vi "Compile EPTx RevA Data.vi"(8 "error in (no error)":errorcluster, 10 "Compiled Data":T1 {"DI-B Injection"."Settings"."Pump Phase Array"."Profile" max=15; "DI-B Injection"."Settings"."Pump Phase Array"."Period [s]" min=0 max=0.000102 format="%#_3p"; "DI-B Injection"."Settings"."Pump Phase Array"."Pulse Width [s]" min=0 max=0.000102 format="%#_3p"; "DI-B Injection"."Settings"."Pump Phase Array"."Voltage Low [V]" min=-250 max=250 format="%#_3p"; "DI-B Injection"."Settings"."Pump Phase Array"."Voltage High [V]" min=-250 max=250 format="%#_3p"; "DI-B Injection"."Settings"."Pump Phase Array"."Current Low [A]" min=-40 max=40 format="%#_3p"; "DI-B Injection"."Settings"."Pump Phase Array"."Current High [A]" min=-40 max=40 format="%#_3p"; "DI-B Injection"."Settings"."Pump Phase Array"."Duration [s]" min=0 max=1.67772 format="%#_3p"; "DI-B Injection"."Settings"."Inj Phase Arrays"."Profile" max=15; "DI-B Injection"."Settings"."Inj Phase Arrays"."Period [s]" min=0 max=0.000102 format="%#_3p"; "DI-B Injection"."Settings"."Inj Phase Arrays"."Pulse Width [s]" min=0 max=0.000102 format="%#_3p"; "DI-B Injection"."Settings"."Inj Phase Arrays"."Voltage Low [V]" min=-250 max=250 format="%#_3p"; "DI-B Injection"."Settings"."Inj Phase Arrays"."Voltage High [V]" min=-250 max=250 format="%#_3p"; "DI-B Injection"."Settings"."Inj Phase Arrays"."Current Low [A]" min=-40 max=40 format="%#_3p"; "DI-B Injection"."Settings"."Inj Phase Arrays"."Current High [A]" min=-40 max=40 format="%#_3p"; "DI-B Injection"."Settings"."Inj Phase Arrays"."Duration [s]" min=0 max=1.67772 format="%#_3p"; "DI-A Injection"."Settings"."Pump Phase Array"."Profile" max=15; "DI-A Injection"."Settings"."Pump Phase Array"."Period [s]" min=0 max=0.000102 format="%#_3p"; "DI-A Injection"."Settings"."Pump Phase Array"."Pulse Width [s]" min=0 max=0.000102 format="%#_3p"; "DI-A Injection"."Settings"."Pump Phase Array"."Voltage Low [V]" min=-250 max=250 format="%#_3p"; "DI-A Injection"."Settings"."Pump Phase Array"."Voltage High [V]" min=-250 max=250 format="%#_3p"; "DI-A Injection"."Settings"."Pump Phase Array"."Current Low [A]" min=-40 max=40 format="%#_3p"; "DI-A Injection"."Settings"."Pump Phase Array"."Current High [A]" min=-40 max=40 format="%#_3p"; "DI-A Injection"."Settings"."Pump Phase Array"."Duration [s]" min=0 max=1.67772 format="%#_3p"; "DI-A Injection"."Settings"."Inj Phase Arrays"."Profile" max=15; "DI-A Injection"."Settings"."Inj Phase Arrays"."Period [s]" min=0 max=0.000102 format="%#_3p"; "DI-A Injection"."Settings"."Inj Phase Arrays"."Pulse Width [s]" min=0 max=0.000102 format="%#_3p"; "DI-A Injection"."Settings"."Inj Phase Arrays"."Voltage Low [V]" min=-250 max=250 format="%#_3p"; "DI-A Injection"."Settings"."Inj Phase Arrays"."Voltage High [V]" min=-250 max=250 format="%#_3p"; "DI-A Injection"."Settings"."Inj Phase Arrays"."Current Low [A]" min=-40 max=40 format="%#_3p"; "DI-A Injection"."Settings"."Inj Phase Arrays"."Current High [A]" min=-40 max=40 format="%#_3p"; "DI-A Injection"."Settings"."Inj Phase Arrays"."Duration [s]" min=0 max=1.67772 format="%#_3p"; "Knock"."Settings"."Sensor Select" items=["Sensor 1", "Sensor 2", "Sensor 3", "Sensor 4", "Sensor 5", "Sensor 6", "Sensor 7", "Sensor 8", "Sensor 9", "Sensor 10", "Sensor 11", "Sensor 12"]; "PBx"."PB-01"."FIFO Indexes"."Read"."UEGO Diagnostics"."LSUType" format="%02.0f"; "PBx"."PB-01"."FIFO Indexes"."Read"."UEGO Diagnostics"."UEGOFuseStatus" format="%02.0f"; "DCM Core"."Settings"."System Settings"."HH Open Threshold [A]" min=0 max=8 format="%#_3p"; "DCM Core"."Settings"."System Settings"."HH ISeq Dur PS" items=["3.3ms @ 20MHz"=0, "6.5ms @ 10MHz"=4, "13ms @ 5MHz"=6, "26ms @ 2.5MHz"=7]; "DCM Core"."Settings"."System Settings"."HH Shoot Through Time [s]" min=0 max=0.003277 format="%#_3p"; "DCM Core"."Settings"."System Settings"."Clamp Fault Filter Time [s]" min=0 max=0.003277 format="%#_3p"; "DCM Core"."Settings"."System Settings"."DI HS Fault Filter Time [s]" min=0 max=0.003277 format="%#_3p"; "DCM Core"."Settings"."B Configuration"."Pump Zener Voltage [V]" min=0 max=240 format="%#_13g"; "DCM Core"."Settings"."B Configuration"."DI Zener Voltage [V]" min=0 max=100 format="%#_13g"; "DCM Core"."Settings"."B Configuration"."Boost Clamp [V]" min=0 max=220 format="%#_13g"; "DCM Core"."Settings"."B Configuration"."Boost Voltage [V]" min=0 max=220 format="%#_13g"; "DCM Core"."Settings"."A Configuration"."Pump Zener Voltage [V]" min=0 max=240 format="%#_13g"; "DCM Core"."Settings"."A Configuration"."DI Zener Voltage [V]" min=0 max=100 format="%#_13g"; "DCM Core"."Settings"."A Configuration"."Boost Clamp [V]" min=0 max=220 format="%#_13g"; "DCM Core"."Settings"."A Configuration"."Boost Voltage [V]" min=0 max=220 format="%#_13g"; "DCM Core"."FIFO Indexes"."Write"."HH Config"."ISeq"."Duration [s]" min=0 max=26; "DCM Core"."FIFO Indexes"."Write"."HH Config"."ISeq"."Lower [A]" min=0 max=8; "DCM Core"."FIFO Indexes"."Write"."HH Config"."ISeq"."Upper [A]" min=0 max=8; "Digital Signals"."Settings"."Aux In Filters [s]" min=0; "Digital Signals"."Settings"."Diff IO Filters [s]" min=0; "EPTx RevA"."Settings"."EPTxFilters"."Aux 4 [s]" format="%#_6p"; "EPTx RevA"."Settings"."EPTxFilters"."Aux 3 [s]" format="%#_6p"; "EPTx RevA"."Settings"."EPTxFilters"."Aux 2 [s]" format="%#_6p"; "EPTx RevA"."Settings"."EPTxFilters"."Aux 1 [s]" format="%#_6p"; "EPTx RevA"."Settings"."EPTxFilters"."Primary [s]" format="%#_6p"}, 11 "Device Item Ref in":T40 format="%.0x") -> (0 "error out":errorcluster, 2 "Compiled Data":T1 {"DI-B Injection"."Settings"."Pump Phase Array"."Profile" max=15; "DI-B Injection"."Settings"."Pump Phase Array"."Period [s]" min=0 max=0.000102 format="%#_3p"; "DI-B Injection"."Settings"."Pump Phase Array"."Pulse Width [s]" min=0 max=0.000102 format="%#_3p"; "DI-B Injection"."Settings"."Pump Phase Array"."Voltage Low [V]" min=-250 max=250 format="%#_3p"; "DI-B Injection"."Settings"."Pump Phase Array"."Voltage High [V]" min=-250 max=250 format="%#_3p"; "DI-B Injection"."Settings"."Pump Phase Array"."Current Low [A]" min=-40 max=40 format="%#_3p"; "DI-B Injection"."Settings"."Pump Phase Array"."Current High [A]" min=-40 max=40 format="%#_3p"; "DI-B Injection"."Settings"."Pump Phase Array"."Duration [s]" min=0 max=1.67772 format="%#_3p"; "DI-B Injection"."Settings"."Inj Phase Arrays"."Profile" max=15; "DI-B Injection"."Settings"."Inj Phase Arrays"."Period [s]" min=0 max=0.000102 format="%#_3p"; "DI-B Injection"."Settings"."Inj Phase Arrays"."Pulse Width [s]" min=0 max=0.000102 format="%#_3p"; "DI-B Injection"."Settings"."Inj Phase Arrays"."Voltage Low [V]" min=-250 max=250 format="%#_3p"; "DI-B Injection"."Settings"."Inj Phase Arrays"."Voltage High [V]" min=-250 max=250 format="%#_3p"; "DI-B Injection"."Settings"."Inj Phase Arrays"."Current Low [A]" min=-40 max=40 format="%#_3p"; "DI-B Injection"."Settings"."Inj Phase Arrays"."Current High [A]" min=-40 max=40 format="%#_3p"; "DI-B Injection"."Settings"."Inj Phase Arrays"."Duration [s]" min=0 max=1.67772 format="%#_3p"; "DI-A Injection"."Settings"."Pump Phase Array"."Profile" max=15; "DI-A Injection"."Settings"."Pump Phase Array"."Period [s]" min=0 max=0.000102 format="%#_3p"; "DI-A Injection"."Settings"."Pump Phase Array"."Pulse Width [s]" min=0 max=0.000102 format="%#_3p"; "DI-A Injection"."Settings"."Pump Phase Array"."Voltage Low [V]" min=-250 max=250 format="%#_3p"; "DI-A Injection"."Settings"."Pump Phase Array"."Voltage High [V]" min=-250 max=250 format="%#_3p"; "DI-A Injection"."Settings"."Pump Phase Array"."Current Low [A]" min=-40 max=40 format="%#_3p"; "DI-A Injection"."Settings"."Pump Phase Array"."Current High [A]" min=-40 max=40 format="%#_3p"; "DI-A Injection"."Settings"."Pump Phase Array"."Duration [s]" min=0 max=1.67772 format="%#_3p"; "DI-A Injection"."Settings"."Inj Phase Arrays"."Profile" max=15; "DI-A Injection"."Settings"."Inj Phase Arrays"."Period [s]" min=0 max=0.000102 format="%#_3p"; "DI-A Injection"."Settings"."Inj Phase Arrays"."Pulse Width [s]" min=0 max=0.000102 format="%#_3p"; "DI-A Injection"."Settings"."Inj Phase Arrays"."Voltage Low [V]" min=-250 max=250 format="%#_3p"; "DI-A Injection"."Settings"."Inj Phase Arrays"."Voltage High [V]" min=-250 max=250 format="%#_3p"; "DI-A Injection"."Settings"."Inj Phase Arrays"."Current Low [A]" min=-40 max=40 format="%#_3p"; "DI-A Injection"."Settings"."Inj Phase Arrays"."Current High [A]" min=-40 max=40 format="%#_3p"; "DI-A Injection"."Settings"."Inj Phase Arrays"."Duration [s]" min=0 max=1.67772 format="%#_3p"; "Knock"."Settings"."Sensor Select" items=["Sensor 1", "Sensor 2", "Sensor 3", "Sensor 4", "Sensor 5", "Sensor 6", "Sensor 7", "Sensor 8", "Sensor 9", "Sensor 10", "Sensor 11", "Sensor 12"]; "PBx"."PB-01"."FIFO Indexes"."Read"."UEGO Diagnostics"."LSUType" format="%02.0f"; "PBx"."PB-01"."FIFO Indexes"."Read"."UEGO Diagnostics"."UEGOFuseStatus" format="%02.0f"; "DCM Core"."Settings"."System Settings"."HH Open Threshold [A]" min=0 max=8 format="%#_3p"; "DCM Core"."Settings"."System Settings"."HH ISeq Dur PS" items=["3.3ms @ 20MHz"=0, "6.5ms @ 10MHz"=4, "13ms @ 5MHz"=6, "26ms @ 2.5MHz"=7]; "DCM Core"."Settings"."System Settings"."HH Shoot Through Time [s]" min=0 max=0.003277 format="%#_3p"; "DCM Core"."Settings"."System Settings"."Clamp Fault Filter Time [s]" min=0 max=0.003277 format="%#_3p"; "DCM Core"."Settings"."System Settings"."DI HS Fault Filter Time [s]" min=0 max=0.003277 format="%#_3p"; "DCM Core"."Settings"."B Configuration"."Pump Zener Voltage [V]" min=0 max=240 format="%#_13g"; "DCM Core"."Settings"."B Configuration"."DI Zener Voltage [V]" min=0 max=100 format="%#_13g"; "DCM Core"."Settings"."B Configuration"."Boost Clamp [V]" min=0 max=220 format="%#_13g"; "DCM Core"."Settings"."B Configuration"."Boost Voltage [V]" min=0 max=220 format="%#_13g"; "DCM Core"."Settings"."A Configuration"."Pump Zener Voltage [V]" min=0 max=240 format="%#_13g"; "DCM Core"."Settings"."A Configuration"."DI Zener Voltage [V]" min=0 max=100 format="%#_13g"; "DCM Core"."Settings"."A Configuration"."Boost Clamp [V]" min=0 max=220 format="%#_13g"; "DCM Core"."Settings"."A Configuration"."Boost Voltage [V]" min=0 max=220 format="%#_13g"; "DCM Core"."FIFO Indexes"."Write"."HH Config"."ISeq"."Duration [s]" min=0 max=26; "DCM Core"."FIFO Indexes"."Write"."HH Config"."ISeq"."Lower [A]" min=0 max=8; "DCM Core"."FIFO Indexes"."Write"."HH Config"."ISeq"."Upper [A]" min=0 max=8; "Digital Signals"."Settings"."Aux In Filters [s]" min=0; "Digital Signals"."Settings"."Diff IO Filters [s]" min=0; "EPTx RevA"."Settings"."EPTxFilters"."Aux 4 [s]" format="%#_6p"; "EPTx RevA"."Settings"."EPTxFilters"."Aux 3 [s]" format="%#_6p"; "EPTx RevA"."Settings"."EPTxFilters"."Aux 2 [s]" format="%#_6p"; "EPTx RevA"."Settings"."EPTxFilters"."Aux 1 [s]" format="%#_6p"; "EPTx RevA"."Settings"."EPTxFilters"."Primary [s]" format="%#_6p"}, 3 "Device Item Ref out":T40 format="%.0x")   [LabVIEW 2016, in "DCM System Explorer.lvlib"]
uses:
  DCM System Explorer.lvlib
  <vilib>/NI Veristand/Custom Device API/Custom Device Item Ref.ctl
  Shared/Types/Compiled Data.ctl
  <vilib>/NI Veristand/Custom Device Waveform API/Multiple Waveforms Write (DBL)/Multiple Waveforms Write (DBL).lvclass
  Shared/Types/Engine Init Data.ctl
  Shared/Types/Engine Status.ctl
  Shared/Types/EPTx RevA RT Data.ctl
  Built/DCM Classes Packed/Pharlap/C/DCM-Classes.lvlibp/1abvi3w/vi.lib/Powertrain Controls/Device Drivers/DCM/Rev0/FPGA/Digital Channel.ctl
  Built/DCM Classes Packed/Pharlap/C/DCM-Classes.lvlibp/Engine Position Tracking/EPTx/RevA/RT/Controls/EPTxFilters.ctl
  Shared/Types/DCM Core.ctl
  Shared/Types/System State Indexes.ctl
  Shared/Types/DI Faults Indexes.ctl
  Shared/Types/HH Status Indexes.ctl
  Shared/Types/HH Config Indexes.ctl
  <vilib>/Powertrain Controls/Device Drivers/DCM/Rev0/RT/Configuration.ctl
  <vilib>/Powertrain Controls/Device Drivers/DCM/Rev0/FPGA/DI - Bank Configuration.ctl
  <vilib>/Powertrain Controls/Device Drivers/DCM/Rev0/RT/System Settings.ctl
  <vilib>/Powertrain Controls/Device Drivers/DCM/Rev0/RT/User LED.ctl
  <vilib>/Powertrain Controls/Device Drivers/DCM/HH/RT/Duration Pre Scale.ctl
  Shared/Types/DI.ctl
  Shared/Types/DI Command Indexes.ctl
  Shared/Types/DI Phase Outputs.ctl
  <vilib>/Powertrain Controls/Device Drivers/DCM/DI/RT/Phase.ctl
  <vilib>/Powertrain Controls/Device Drivers/DCM/Rev0/FPGA/DI - Drive State.ctl
  <vilib>/Powertrain Controls/Device Drivers/DCM/DI/FPGA/Phase Step.ctl
  <vilib>/Powertrain Controls/Device Drivers/DCM/DI/FPGA/Control.ctl
  Shared/Types/DiffIO.ctl
  Shared/Types/DiffIO Results Indexes.ctl
  Shared/Types/DiffIO Setup Indexes.ctl
  Shared/Types/HH.ctl
  Shared/Types/HH Command Indexes.ctl
  Shared/Types/DI Scope.ctl
  <vilib>/NI Veristand/Custom Device API/Waveform Data Reference.ctl
  Shared/Types/HH Scope.ctl
  Shared/Types/Digital Signals.ctl
  Shared/Types/Skip Fire.ctl
  Shared/Types/Skip Fire Setup Indexes.ctl
  Shared/Types/Knock.ctl
  Shared/Types/PBx.ctl
  Shared/Types/PB-01.ctl
  Shared/Types/ESTTL Setup Indexes.ctl
  <vilib>/Powertrain Controls/Device Drivers/VR-Hall/RevC/Real-Time/Support/Vr_Hall_mode_control_revc.ctl
  Shared/Types/EPTx Signal Select.ctl
  <vilib>/Powertrain Controls/Device Drivers/DCM/Rev0/FPGA/Digital Channel.ctl
  Shared/Types/EPTx RevA RT Configuration.ctl
  <vilib>/Powertrain Controls/Device Drivers/Engine Position Tracking/EPTx/RevA/RT/Controls/EPTxFilters.ctl
  Shared/DCM Properties.vi
  Shared/DCM Constants and GUIDs.vi
  <vilib>/NI Veristand/Custom Device Tools/Custom Device Utility Library/NI VeriStand - Search for Item by GUID.vi
  <vilib>/NI Veristand/Custom Device Tools/Custom Device Utility Library/Custom Device Utility Library.lvlib
  DCM Shared.lvlib
  <vilib>/Powertrain Controls/Device Drivers/DCM/Rev0/FPGA/DCM - FPGA.lvlib
  <vilib>/Powertrain Controls/Device Drivers/Engine Position Tracking/EPTx/RevA/RT/EPTx - RevA - RT.lvlib
  <vilib>/NI VeriStand/Custom Device API/Custom Device API.lvlib
  <vilib>/Powertrain Controls/Device Drivers/DCM/Rev0/RT/DCM - RT.lvclass
  <vilib>/Powertrain Controls/Device Drivers/DCM/HH/RT/DCM - RT - HH.lvlib
  <vilib>/Powertrain Controls/Device Drivers/DCM/DI/FPGA/DCM - FPGA - DI.lvlib
  <vilib>/Powertrain Controls/Device Drivers/DCM/DI/RT/DCM - RT - DI.lvlib
  Built/DCM Classes Packed/Pharlap/C/DCM-Classes.lvlibp/Engine Position Tracking/EPTx/RevA/RT/EPTx - RevA - RT.lvlib
  Built/DCM Classes Packed/Pharlap/C/DCM-Classes.lvlibp/1abvi3w/vi.lib/Powertrain Controls/Device Drivers/DCM/Rev0/FPGA/DCM - FPGA.lvlib
panel:
  # "Voltage [DV]"
  # "Voltage [V]"
  # "Voltage [DV]"
  # "Voltage [V]"
  # "Voltage [DV]"
  # "Voltage [V]"
  # "Voltage [DV]"
  # "Voltage [V]"
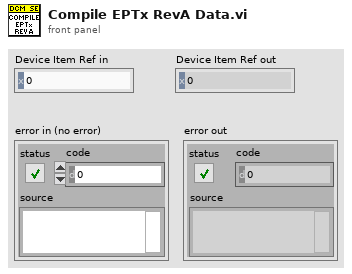
[diagram p1: front panel]
types:
  T1 = typedef "DCM Shared.lvlib/Compiled Data.ctl" = cluster{"Init":T2, "Cmd Status":T3, "Sys Status":T3, "EPTx RevA":T4, "DCM Core":T7, "DI-A Injection":T17, "DI-B Injection":T17, "DiffIO":T24, "HH Cmd":T27, "DI ADC":T29, "HH ADC":T31, "Digital Signals":T32, "Skip Fire":T33, "Knock":T35, "PBx":T36}
  T2 = typedef "DCM Shared.lvlib/Engine Init Data.ctl" = cluster{"Name":string, "RIO Address":string, "Bitfile Path RT":path, "Username":string, "Password":string, "Cmd CPU":i32, "Cmd Decimation":i32, "Cmd Priority":i32, "Sys CPU":i32, "Sys Decimation":i32, "Sys Priority":i32, "Input FIFO Size":i32, "Output FIFO Size":i32, "Compile Time":dbl}
  T3 = typedef "DCM Shared.lvlib/Engine Status.ctl" = cluster{"FIFO indexes":cluster{"code":i32, "loop duration":i32, "late count":i32}}
  T4 = typedef "DCM Shared.lvlib/EPTx RevA RT Data.ctl" = cluster{"FIFO Indexes":cluster{"Read":cluster{"Sync":i32, "CurrentCAD":i32, "Speed":i32, "Config":i32, "Rcvg Primary":i32, "Stall":i32, "Overflow Error":i32, "Ratio Error":i32, "Pattern Error":i32, "Aux Warning":i32, "Watchdog Error":i32, "Loading":i32}, "Write":cluster{"Reload EPTx":i32, "Sync Enable":i32, "Clear Errors":i32, "Sim Enable":i32, "Sim Speed":i32}}, "Settings":cluster{"EPTxConfigFilename":string, "EPTx Signal Select":cluster{"Primary":T5, "Aux 1":T5, "Aux 2":T5, "Aux 3":T5, "Aux 4":T5}, "FPGAFrequency":sgl, "StallSpeed":sgl, "EPTxFilters":T6, "History":u8}}
  T5 = typedef "DCM-Classes.lvlibp/DCM - FPGA.lvlib/Digital Channel.ctl" = enum8{"Unused", "User OS", "Diff IO 1", "Diff IO 2", "Diff IO 3", "Diff IO 4", "Diff IO 5", "Diff IO 6", "Diff IO 7", "Diff IO 8", "Aux 1", "Aux 2", "Aux 3", "Aux 4", "Aux 5", "Aux 6", "Aux 7", "Aux 8", "Aux 9", "Aux 10", "Aux 11", "Aux 12", "Aux 13", "Aux 14", "Aux 15", "Aux 16"}
  T6 = typedef "DCM-Classes.lvlibp/EPTx - RevA - RT.lvlib/EPTxFilters.ctl" = cluster{"Primary [s]":sgl, "Aux 1 [s]":sgl, "Aux 2 [s]":sgl, "Aux 3 [s]":sgl, "Aux 4 [s]":sgl}
  T7 = typedef "DCM Shared.lvlib/DCM Core.ctl" = cluster{"FIFO Indexes":cluster{"A Run State":i32, "B Run State":i32, "Read":cluster{"Status":T8, "A DI Faults":T9[], "B DI Faults":T9[], "HH Status":T10[]}, "Write":cluster{"A Config":cluster{"PowerSupplyEnable":i32, "InjectEnable":i32, "BoostVoltage":i32}, "B Config":cluster{"PowerSupplyEnable":i32, "InjectEnable":i32, "BoostVoltage":i32}, "HH Config":T11[], "System Settings":cluster{"MPRD":i32, "UserLED1":i32, "UserLED2":i32}, "A Fault Clear":cluster{"1":i32, "2":i32, "3":i32, "4":i32, "5":i32, "6":i32, "7":i32, "8":i32}, "B Fault Clear":cluster{"1":i32, "2":i32, "3":i32, "4":i32, "5":i32, "6":i32, "7":i32, "8":i32}}}, "Settings":cluster{"A Configuration":T12, "B Configuration":T12, "System Settings":T14}}
  T8 = typedef "DCM Shared.lvlib/System State Indexes.ctl" = cluster{"System ADC":cluster{"AI 1 [V]":i32, "AI 2 [V]":i32, "AI 3 [V]":i32, "AI 4 [V]":i32, "AI 5 [V]":i32, "AI 6 [V]":i32, "AI 7 [V]":i32, "AI 8 [V]":i32, "AI 9 [V]":i32, "AI 10 [V]":i32, "AI 11 [V]":i32, "AI 12 [V]":i32, "Temp HH 1-6 [C]":i32, "Temp HH 7-12 [C]":i32, "Temp DI A [C]":i32, "Temp DI Zener A [C]":i32, "Temp DI B [C]":i32, "Temp DI Zener B [C]":i32, "Temp CPU [C]":i32, "Temp Fan Intake [C]":i32, "Temp Secondary A [C]":i32, "Temp Primary A [C]":i32, "Temp Boost B [C]":i32, "Primary Range [V]":i32, "Primary A1A2 [V]":i32, "Primary A3A4 [V]":i32, "Primary B3B4 [V]":i32, "Primary B1B2 [V]":i32, "Secondary A1A2 [V]":i32, "Secondary A3A4 [V]":i32, "Secondary B3B4 [V]":i32, "Secondary B1B2 [V]":i32, "Ext HV A [V]":i32, "Ext HV B [V]":i32, "FET Driver [V]":i32, "Fan [V]":i32, "Battery [V]":i32, "DRVP [V]":i32, "Key [V]":i32, "DI Zener A [V]":i32, "DI Zener B [V]":i32, "Pump Zener A [V]":i32, "Pump Zener B [V]":i32, "MPRD [V]":i32}, "IO Lock":i32, "HH Mode Config Error":i32, "Fan Speed 1 [RPM]":i32, "Fan Speed 2 [RPM]":i32, "Firmware Major Rev":i32, "Firmware Minor Rev":i32, "Internal Fault":i32, "Fault Value":i32}
  T9 = typedef "DCM Shared.lvlib/DI Faults Indexes.ctl" = cluster{"HV Fault":i32, "LV Fault":i32, "LS Fault":i32, "MUX Fault":i32, "Open Warning":i32}
  T10 = typedef "DCM Shared.lvlib/HH Status Indexes.ctl" = cluster{"Current [A]":i32, "Config Error":i32, "Short Fault":i32, "Open Fault":i32, "Period Min [A]":i32, "Period Max [A]":i32, "Period Avg [A]":i32, "On Avg [A]":i32}
  T11 = typedef "DCM Shared.lvlib/HH Config Indexes.ctl" = cluster{"Mode":i32, "IO Lock State":i32, "Phase 1 FP":i32, "Fault Clear":i32, "ISeq":cluster{"Upper [A]":i32, "Lower [A]":i32, "Duration [s]":i32}[]}
  T12 = typedef "DCM - RT.lvclass/Configuration.ctl" = cluster{"Configuration":T13, "Power Supply Enable":bool, "Boost Voltage [V]":sgl, "Inject Enable":bool, "DI Zener Enable":bool, "DI Zener Voltage [V]":sgl, "Pump Zener Enable":bool, "Pump Zener Voltage [V]":sgl, "Boost Clamp [V]":sgl}
  T13 = typedef "DCM - FPGA.lvlib/DI - Bank Configuration.ctl" = enum8{"Solenoid Unipolar 4", "Solenoid Unipolar 7 (Muxed)", "Solenoid Unipolar 8 (Muxed)", "Solenoid Bipolar 2", "Solenoid Bipolar 3 (Muxed)", "Piezo Unipolar 2", "Piezo Unipolar 3 (Muxed)", "Piezo Unipolar 4 (Muxed)", "Piezo Bipolar 2", "Piezo Bipolar 3 (Muxed)"}
  T14 = typedef "DCM - RT.lvclass/System Settings.ctl" = cluster{"MPRD":bool, "IO Lock MPRD Disable":bool, "User LED 1":T15, "User LED 2":T15, "DI HS Fault Filter Time [s]":sgl, "Clamp Fault Filter Time [s]":sgl, "HH Shoot Through Time [s]":sgl, "HH ISeq Dur PS":T16, "HH Open Threshold [A]":sgl}
  T15 = typedef "DCM - RT.lvclass/User LED.ctl" = enum16{"Off", "Yellow", "Green"}
  T16 = typedef "DCM - RT - HH.lvlib/Duration Pre Scale.ctl" = u8
  T17 = typedef "DCM Shared.lvlib/DI.ctl" = cluster{"DI Command Enabled":bool, "Sync Pump Enabled":bool, "FIFO Indexes":cluster{"Write":cluster{"DI Command":T18[], "Pump Command":T18}}, "Settings":T19}
  T18 = typedef "DCM Shared.lvlib/DI Command Indexes.ctl" = cluster{"Mode":i32, "Digital Input":i32, "Default Profile Index":i32, "Cal Freq [Hz]":i32, "Cal Duration [s]":i32, "Cal Increment [s]":i32, "Cal Pulses":i32, "TMP Command Sequence":cluster{"Duration [s]":i32, "Level":i32, "Run/Stop":i32, "Profile Index":i32}[], "EPT TDC Offset [CAD]":i32, "EPT Window Start [DBTDC]":i32, "EPT Window End [DBTDC]":i32, "EPT Angles":cluster{"Enable":i32, "Timing [DBTDC]":i32, "Duration [s]":i32, "Profile Index":i32}[], "EPT Skip Fire":i32, "EPT Skip Index":i32, "EPT Precharge Duration [s]":i32, "EPT Precharge Profile Index":i32}
  T19 = typedef "DCM Shared.lvlib/DI Phase Outputs.ctl" = cluster{"Inj Phase Arrays":T20[][], "Pump Phase Array":T20[], "Pulsewidths [s]":sgl[][]}
  T20 = typedef "DCM - RT - DI.lvlib/Phase.ctl" = cluster{"Drive":T21, "Direction":bool, "Phase Step":T22, "Duration [s]":sgl, "Current High [A]":sgl, "Current Low [A]":sgl, "Voltage High [V]":sgl, "Voltage Low [V]":sgl, "Change":bool, "Current Control":T23, "Period [s]":sgl, "Pulse Width [s]":sgl, "Profile":u8, "Voltage Control":bool}
  T21 = typedef "DCM - FPGA.lvlib/DI - Drive State.ctl" = enum8{"Idle", "HV Current Control", "LV Current Control", "Back Boost", "Piezo Charge", "Piezo Discharge"}
  T22 = typedef "DCM - FPGA - DI.lvlib/Phase Step.ctl" = enum8{"Duration", "First Peak", "End of Cmd", "Branch", "2-Phase Duration"}
  T23 = typedef "DCM - FPGA - DI.lvlib/Control.ctl" = enum8{"Closed Loop", "Fixed Period", "Fixed On Pulse", "Fixed Off Pulse", "Open Loop", "Profile"}
  T24 = typedef "DCM Shared.lvlib/DiffIO.ctl" = cluster{"DiffIO Command Enabled":bool, "FIFO Indexes":cluster{"Read":cluster{"Diff IO Results":T25[], "DiffIOIn":cluster{"1":i32, "2":i32, "3":i32, "4":i32, "5":i32, "6":i32, "7":i32, "8":i32}}, "Write":cluster{"Diff I/O Setup":T26[]}}}
  T25 = typedef "DCM Shared.lvlib/DiffIO Results Indexes.ctl" = cluster{"Capture [DBTDC]":i32, "Capture Error":i32, "Frequency [Hz]":i32, "Duty Cycle [%]":i32, "PWM Stopped":i32}
  T26 = typedef "DCM Shared.lvlib/DiffIO Setup Indexes.ctl" = cluster{"Mode":i32, "Capture Start [DBTDC]":i32, "Capture End [DBTDC]":i32, "Polarity":i32, "Frequency [Hz]":i32, "Duty Cycle [%]":i32, "TDC Offset [CAD]":i32, "Window Start [DBTDC]":i32, "Window End [DBTDC]":i32, "Angles":cluster{"Enable":i32, "Location [DBTDC]":i32, "Duration [s]":i32}[], "Skip Fire":i32, "Skip Fire Index":i32}
  T27 = typedef "DCM Shared.lvlib/HH.ctl" = cluster{"HH Command Enabled":bool, "FIFO Indexes":cluster{"Write":T28[]}}
  T28 = typedef "DCM Shared.lvlib/HH Command Indexes.ctl" = cluster{"Mode":i32, "Digital Input":i32, "Polarity":i32, "Frequency [Hz]":i32, "Duty Cycle [%]":i32, "TDC Offset [CAD]":i32, "Window Start [DBTDC]":i32, "Window End [DBTDC]":i32, "Angles":cluster{"Enable":i32, "Location [DBTDC]":i32, "Duration [s]":i32}[], "Skip Fire":i32, "Skip Fire Index":i32}
  T29 = typedef "DCM Shared.lvlib/DI Scope.ctl" = cluster{"FIFO Indexes":cluster{"Write":cluster{"Capture Enable":i32, "Capture Event":i32, "Capture Length":i32, "DI ADC 1 Select":i32, "DI ADC 2 Select":i32, "DI ADC 3 Select":i32, "DI ADC 4 Select":i32}, "Read":cluster{"Capture dt [s]":i32}}, "DI ADC Data":cluster{"Output Array":sgl[][], "New Data":bool}, "Waveform Data":T30[], "Waveform Session":refnum<class "Multiple Waveforms Write (DBL).lvclass">}
  T30 = typedef "Custom Device API.lvlib/Waveform Data Reference.ctl" = i32
  T31 = typedef "DCM Shared.lvlib/HH Scope.ctl" = cluster{"FIFO Indexes":cluster{"Write":cluster{"Capture Enable":i32, "Capture Event":i32, "Capture Length":i32}, "Read":cluster{"Capture dt [s]":i32}}, "HH ADC Data":cluster{"Output Array":sgl[][], "New Data":bool}, "Waveform Data":T30[], "Waveform Session":refnum<class "Multiple Waveforms Write (DBL).lvclass">}
  T32 = typedef "DCM Shared.lvlib/Digital Signals.ctl" = cluster{"FIFO Indexes":cluster{"Write":cluster{"User OS":i32, "User OS Time [s]":i32}}, "Settings":cluster{"Diff IO Filters [s]":sgl[], "Aux In Filters [s]":sgl[]}}
  T33 = typedef "DCM Shared.lvlib/Skip Fire.ctl" = cluster{"Skip Fire Enabled":bool, "FIFO Indexes":cluster{"Write":cluster{"Setup":T34[]}}}
  T34 = typedef "DCM Shared.lvlib/Skip Fire Setup Indexes.ctl" = cluster{"Enable":i32, "Total Cycles":i32, "On Cycles":i32, "TDC Offset [CAD]":i32}
  T35 = typedef "DCM Shared.lvlib/Knock.ctl" = cluster{"FIFO Indexes":cluster{"Read":cluster{"Knock":i32[], "Knock Intensity":i32[]}, "Write":cluster{"Low Cutoff [Hz]":i32, "High Cutoff [Hz]":i32, "Threshold":i32, "Knock Start [CAD]":i32, "Knock End [CAD]":i32, "Reference Start [CAD]":i32, "Reference End [CAD]":i32}}, "Settings":cluster{"Sensor Select":i32[], "Cylinder Offset [CAD]":sgl[]}}
  T36 = typedef "DCM Shared.lvlib/PBx.ctl" = cluster{"PB Version":u8, "PB-01":T37}
  T37 = typedef "DCM Shared.lvlib/PB-01.ctl" = cluster{"FIFO Indexes":cluster{"Write":cluster{"Clear Faults":i32, "ESTTL Setup":T38[], "UEGO Control":cluster{"UEGO1Enable":i32, "UEGO2Enable":i32, "UEGO1Range":i32, "UEGO2Range":i32, "FilterCutoff (Hz)":i32}}, "Read":cluster{"UEGO Sensor Results":cluster{"UEGO1Lambda":i32, "UEGO1Phi":i32, "UEGO1AFRatio":i32, "UEGO1Ip (mA)":i32, "UEGO2Lambda":i32, "UEGO2Phi":i32, "UEGO2AFRatio":i32, "UEGO2Ip (mA)":i32}, "UEGO Temperature (C)":cluster{"UEGO1Temp (C)":i32, "UEGO2Temp (C)":i32, "UEGO1Hot":i32, "UEGO2Hot":i32}, "UEGO Diagnostics":cluster{"UEGO1SensorFault":i32, "UEGO2SensorFault":i32, "UEGO1HeaterFault":i32, "UEGO2HeaterFault":i32, "UEGOFuseStatus":i32, "Battery (V)":i32, "LSUType":i32}}}, "Settings":cluster{"VR-Hall Mode Select":T39[], "VR-Hall Arming Threshold [V]":dbl[], "ESTTL Command Enabled":bool}}
  T38 = typedef "DCM Shared.lvlib/ESTTL Setup Indexes.ctl" = cluster{"Mode":i32, "Polarity":i32, "Frequency [Hz]":i32, "Duty Cycle [%]":i32, "TDC Offset [CAD]":i32, "Window Start [DBTDC]":i32, "Window End [DBTDC]":i32, "Angles":cluster{"Enable":i32, "Location [DBTDC]":i32, "Duration [s]":i32}[], "Skip Fire":i32, "Skip Fire Index":i32}
  T39 = typedef "Vr_Hall_mode_control_revc.ctl" = enum32{"VR Adaptive Arm", "VR Manual Arm", "Hall", "Hall w/ Pull-up"}
  T40 = typedef "Custom Device API.lvlib/Custom Device Item Ref.ctl" = u64
  T41 = typedef "DCM Shared.lvlib/EPTx RevA RT Configuration.ctl" = cluster{"EPTx Configuration Filename":string, "StallSpeed":dbl, "HistoryCAD":u8, "EPTxFilters":T42}
  T42 = typedef "EPTx - RevA - RT.lvlib/EPTxFilters.ctl" = cluster{"Primary [s]":sgl, "Aux 1 [s]":sgl, "Aux 2 [s]":sgl, "Aux 3 [s]":sgl, "Aux 4 [s]":sgl}
  T43 = typedef "DCM Shared.lvlib/EPTx Signal Select.ctl" = cluster{"Primary":T44, "Aux 1":T44, "Aux 2":T44, "Aux 3":T44, "Aux 4":T44}
  T44 = typedef "DCM - FPGA.lvlib/Digital Channel.ctl" = enum8{"Unused", "User OS", "Diff IO 1", "Diff IO 2", "Diff IO 3", "Diff IO 4", "Diff IO 5", "Diff IO 6", "Diff IO 7", "Diff IO 8", "Aux 1", "Aux 2", "Aux 3", "Aux 4", "Aux 5", "Aux 6", "Aux 7", "Aux 8", "Aux 9", "Aux 10", "Aux 11", "Aux 12", "Aux 13", "Aux 14", "Aux 15", "Aux 16"}
  T45 = typedef "DCM Shared.lvlib/Channel.ctl" = cluster{"Name":string, "Units":string, "Default":dbl, "Description":string}
  T46 = cluster{"FIFO indexes[0]":i32, "FIFO indexes[1]":i32, "FIFO indexes[2]":i32, "FIFO indexes[3]":i32, "FIFO indexes[4]":i32, "FIFO indexes[5]":i32, "FIFO indexes[6]":i32, "FIFO indexes[7]":i32, "FIFO indexes[8]":i32, "FIFO indexes[9]":i32, "FIFO indexes[10]":i32, "FIFO indexes[11]":i32}
  T47 = cluster{"FIFO indexes[0]":i32, "FIFO indexes[1]":i32, "FIFO indexes[2]":i32, "FIFO indexes[3]":i32, "FIFO indexes[4]":i32}
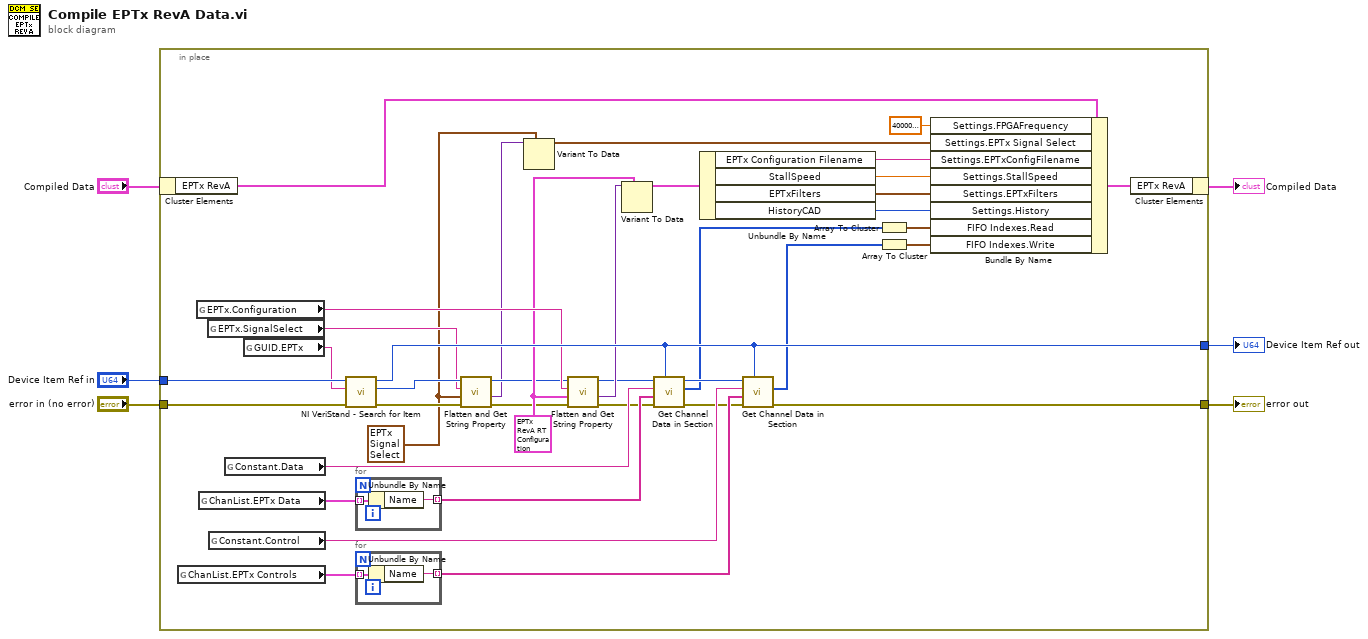
[diagram p0: block diagram]
diagram:
  n1 = in-place {
    in-place-border: "error in (no error)" -> [w44]
    in-place-border: "Device Item Ref in" -> [w43]
    in-place-border: [w41] -> w4
    in-place-border: [w40] -> w3
    w26 = T41 {"EPTx Configuration Filename"="4Str_60m2_Lvl.EPTx", "StallSpeed"=200.0, "HistoryCAD"=63, "EPTxFilters"={"Primary [s]"=0.0, "Aux 1 [s]"=0.0, "Aux 2 [s]"=0.0, "Aux 3 [s]"=0.0, "Aux 4 [s]"=0.0}} ("EPTx Configuration")
    w10 = T43 {"Primary"=enum."Unused", "Aux 1"=enum."Unused", "Aux 2"=enum."Unused", "Aux 3"=enum."Unused", "Aux 4"=enum."Unused"} ("Settings.EPTx Signal Select")
    n2 = in-place-cluster #1("Compiled Data") -> ("EPTx RevA"=w7:T4)
    n3 = global read "DCM Constants and GUIDs.vi" "ChanList.EPTx Controls"() -> (w33:T45[])
    n4 = global read "DCM Properties.vi" "EPTx.Configuration"() -> (w35:string)
    n5 = global read "DCM Constants and GUIDs.vi" "ChanList.EPTx Data"() -> (w34:T45[])
    n6 = global read "DCM Properties.vi" "EPTx.SignalSelect"() -> (w13:string)
    n7 = global read "DCM Constants and GUIDs.vi" "Constant.Control"() -> (w36:string)
    n8 = global read "DCM Constants and GUIDs.vi" "Constant.Data"() -> (w37:string)
    n9 = global read "DCM Constants and GUIDs.vi" "GUID.EPTx"() -> (w42:string)
    n10 = call-poly <vilib>:"NI VeriStand - Search for Item.vi"("error in"=w44, "Item GUID"=w42, "Section Ref in"=w43) -> ("error out"=w18:errorcluster, "Item Ref"=w16:T40, "Section Ref out"=w40:T40)  [unwired: 5 in, 1 out]
    n11 = for {
      tunnel: w34 -> [w48] mode=indexing
      tunnel: [w47] -> w39 mode=indexing
      n12 = Unbundle By Name(w48) -> ("Name"=w47:string)
    }
    n13 = for {
      tunnel: w33 -> [w46] mode=indexing
      tunnel: [w45] -> w38 mode=indexing
      n14 = Unbundle By Name(w46) -> ("Name"=w45:string)
    }
    n15 = call "Flatten and Get String Property.vi"("error in (no error)"=w18, "Default Value"=w10, "Property Name"=w13, "Section Ref in"=w16) -> ("error out"=w17:errorcluster, "Value"=w14:variant, "Section Ref out"=w15:T40)  [unwired: 5 in]
    n16 = Variant To Data(type=w10, Variant=w14) -> (data=w9:T43)  [unwired: 1 in, 1 out]
    n17 = call "Flatten and Get String Property.vi"("error in (no error)"=w17, "Default Value"=w26, "Property Name"=w35, "Section Ref in"=w15) -> ("error out"=w11:errorcluster, "Value"=w25:variant, "Section Ref out"=w12:T40)  [unwired: 5 in]
    n18 = Variant To Data(type=w26, Variant=w25) -> (data=w24:T41)  [unwired: 1 in, 1 out]
    n19 = call "Get Channel Data in Section.vi"("Custom device ref"=w40, "error in (no error)"=w11, "Channels"=w39, "Section (\"\":none)"=w37, "Item Ref in"=w12) -> ("error out"=w32:errorcluster, "FIFO indexes"=w30:i32[], "Item Ref out"=w31:T40)  [unwired: 2 in, 2 out]
    n20 = Unbundle By Name(w24) -> ("EPTx Configuration Filename"=w23:string, "StallSpeed"=w22:dbl, "EPTxFilters"=w21:T42, "HistoryCAD"=w20:u8)
    n21 = call "Get Channel Data in Section.vi"("Custom device ref"=w40, "error in (no error)"=w32, "Channels"=w38, "Section (\"\":none)"=w36, "Item Ref in"=w31) -> ("error out"=w41:errorcluster, "FIFO indexes"=w29:i32[])  [unwired: 2 in, 3 out]
    n22 = Array To Cluster(array=w30) -> (cluster=w28:T46)
    n23 = Array To Cluster(array=w29) -> (cluster=w27:T47)
    n24 = Bundle By Name(cluster=w7, "Settings.FPGAFrequency"=sgl 40000000.0 ("settings.FPGAFrequency"), "Settings.EPTx Signal Select"=w9, "Settings.EPTxConfigFilename"=w23, "Settings.StallSpeed"=w22, "Settings.EPTxFilters"=w21, "Settings.History"=w20, "FIFO Indexes.Read"=w28, "FIFO Indexes.Write"=w27) -> (w8:T4)
    n25 = in-place-cluster #1("EPTx RevA"=w8) -> (→"Compiled Data":T1)
  }
  "error out" <- w4
  "Device Item Ref out" <- w3
